vi "getOffsetToTAI.vi"(10 "Epoch Time":i64=2272060800, 11 "Epoch.GPS":refnum<class "Epoch.GPS.lvclass">) -> (2 "Offset to TAI":i64)   [LabVIEW 2013, in "Epoch.GPS.lvclass"]
uses:
  Epoch.GPS.lvclass
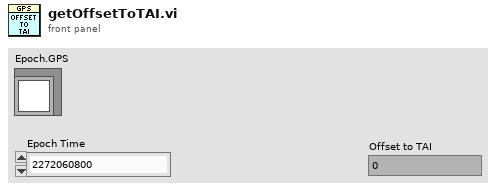
[diagram p1: front panel]
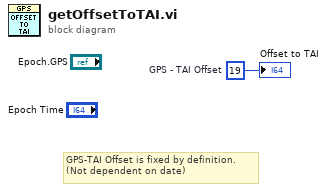
[diagram p0: block diagram]
diagram:
  w1 = i64 19  # GPS - TAI Offset
  # "GPS-TAI Offset is fixed by definition.\n(Not dependent on date)"
  "Offset to TAI" <- w1
